vi "Build Number Name.vi"(10 "Base File Name":string, 11 "File #":u32) -> (2 "Numbered Name":string)   [LabVIEW 2014, in "TDMS Logger.lvlib" / "TDMS Logger.lvclass"]
uses:
  TDMS Logger.lvclass
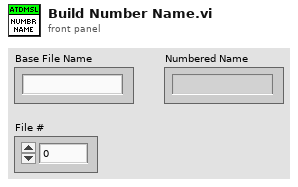
[diagram p1: front panel]
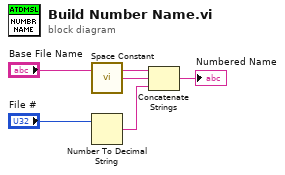
[diagram p0: block diagram]
diagram:
  n1 = call <vilib>:"Space Constant.vi"() -> ("String"=w4:string)
  n2 = Number To Decimal String(number="File #") -> (decimal integer string=w2:string)  [unwired: 1 in]
  n3 = Concatenate Strings("Base File Name", w4, w2) -> (→"Numbered Name":string)
